vi "TiePie.Scp.ScpGetData2Ch.vi"(0 "GenHandle":T1, 1 "qwSampleCount":u64, 2 "qwStartIndex":u64, 3 "pBufferCh1":u64, 4 "pBufferCh2":u64, 5 "error in (no error)":errorcluster) -> (14 "GenHandle out":T1, 15 "data":u64, 19 "error out":errorcluster)   [LabVIEW 2013, in "LVTiePie.lvlib"]
uses:
  LVTiePie.lvlib
  PAN/LabVEW/Tie Pie/bin/libtiepie.dll
  TiePie.Gen.handle.ctl
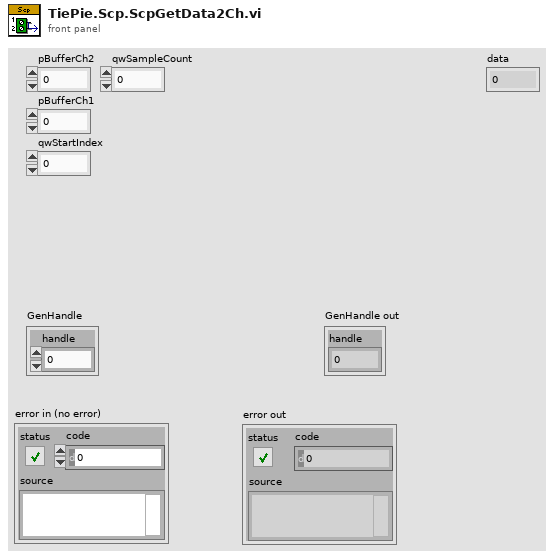
[diagram p1: front panel]
types:
  T1 = typedef "TiePie.Gen.handle.ctl" = cluster{"handle":u32}
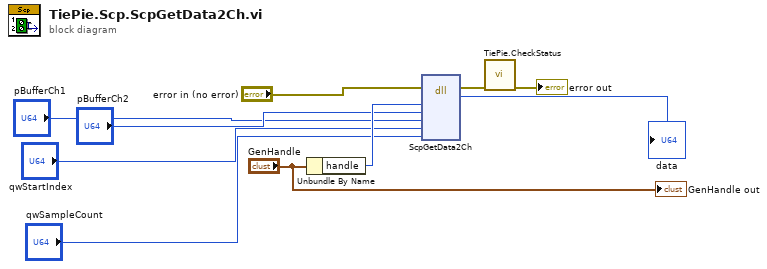
[diagram p0: block diagram]
diagram:
  n1 = Unbundle By Name("GenHandle") -> ("handle"=w9:u32)
  n2 = dll-call lib="C:/Users/mbirski/Desktop/PAN/LabVEW/Tie Pie/bin/libtiepie.dll" fn="ScpGetData2Ch"(error in="error in (no error)", "handle"=w9, "pBufferCh2"="pBufferCh2", "pBufferCh1"="pBufferCh1", "qwStartIndex"="qwStartIndex", "qwSampleCount"="qwSampleCount") -> (error out=w7:errorcluster, "data"=→"data":u64)  [unwired: 7 in, 1 out]
  n3 = call "TiePie.CheckStatus.vi"("error in (no error)"=w7) -> ("error out"=→"error out":errorcluster)  [unwired: 10 in]
  "GenHandle out" <- "GenHandle"
